vi "stage-field-test.vi"() -> ()   [LabVIEW 2014]
uses:
  stage-controller-globals.vi
panel:
  in  "Z max":dbl=200.0
  out "Current Z (um)":ext
  in  "Current Z 2":ext(slide) scale=-1.0..1.0 scale format="%_3f"
  in  "Field Size":enum16{"0", "1", "4", "9", "16"}(ring)=enum."16"
  in  "Field Number":u32(slide)=6 min=1 max=16 step=1 scale=1.0..16.0
  in  "Stop":bool
  in  "Reset":bool
  out "Current (X,Y)":cluster{ext[], ext[]}[](graph)=[{[100.0], [100.0]}, {[100.0, 150.0], [50.0, 50.0]}, {[100.0, 150.0], [100.0, 100.0]}]
  out "At limit 2":bool
  out "At limit":bool
  out "Current X":dbl=100.0 format="%#_13g"
  out "Current Y":dbl=100.0 format="%#_13g"
  in  "x,y step (um)":ext=10.0 format="%_5g"
  in  "x-":bool=TRUE
  in  "x+":bool=TRUE
  in  "y-":bool=TRUE
  in  "y+":bool=TRUE
  in  "Y max":dbl=200.0
  in  "X max":dbl=200.0
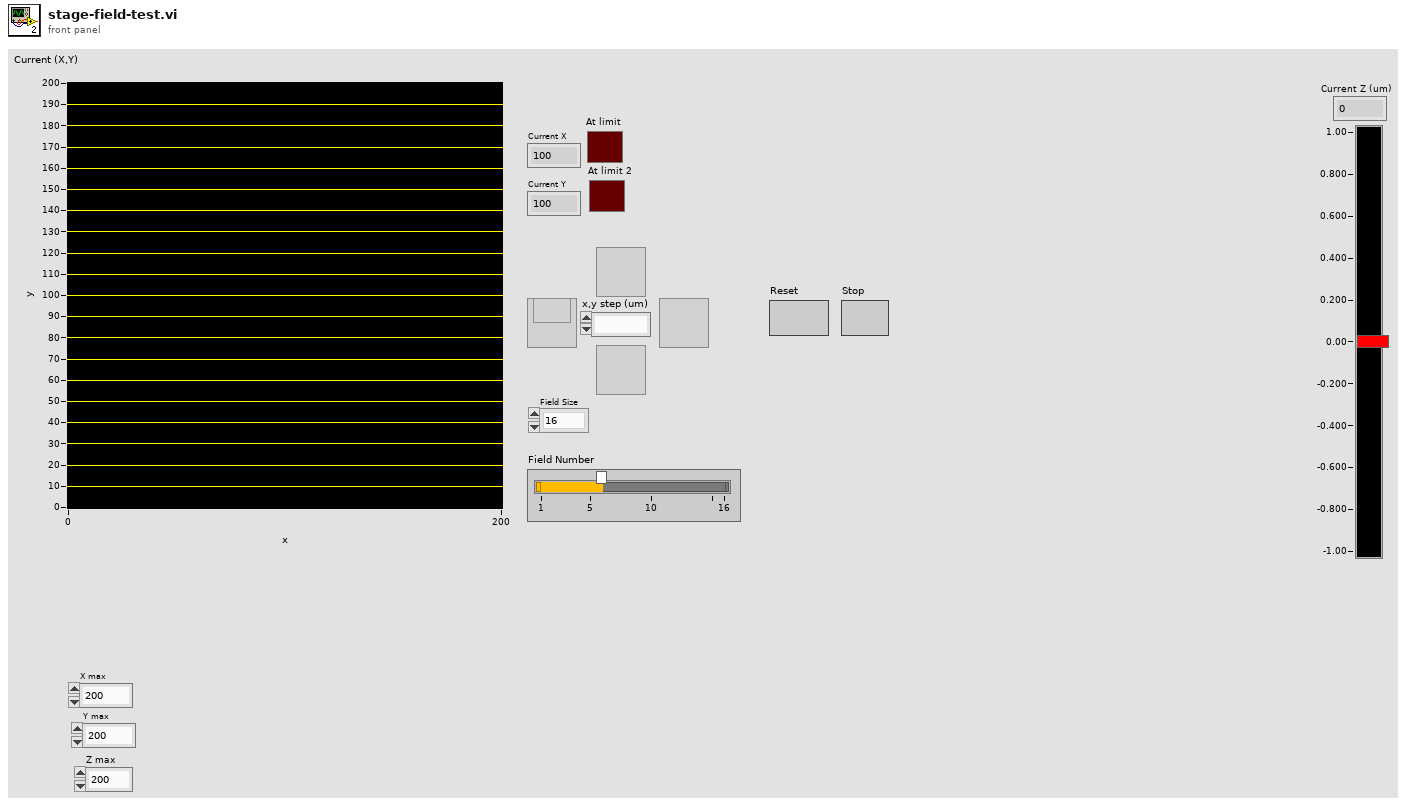
[diagram p1: front panel]
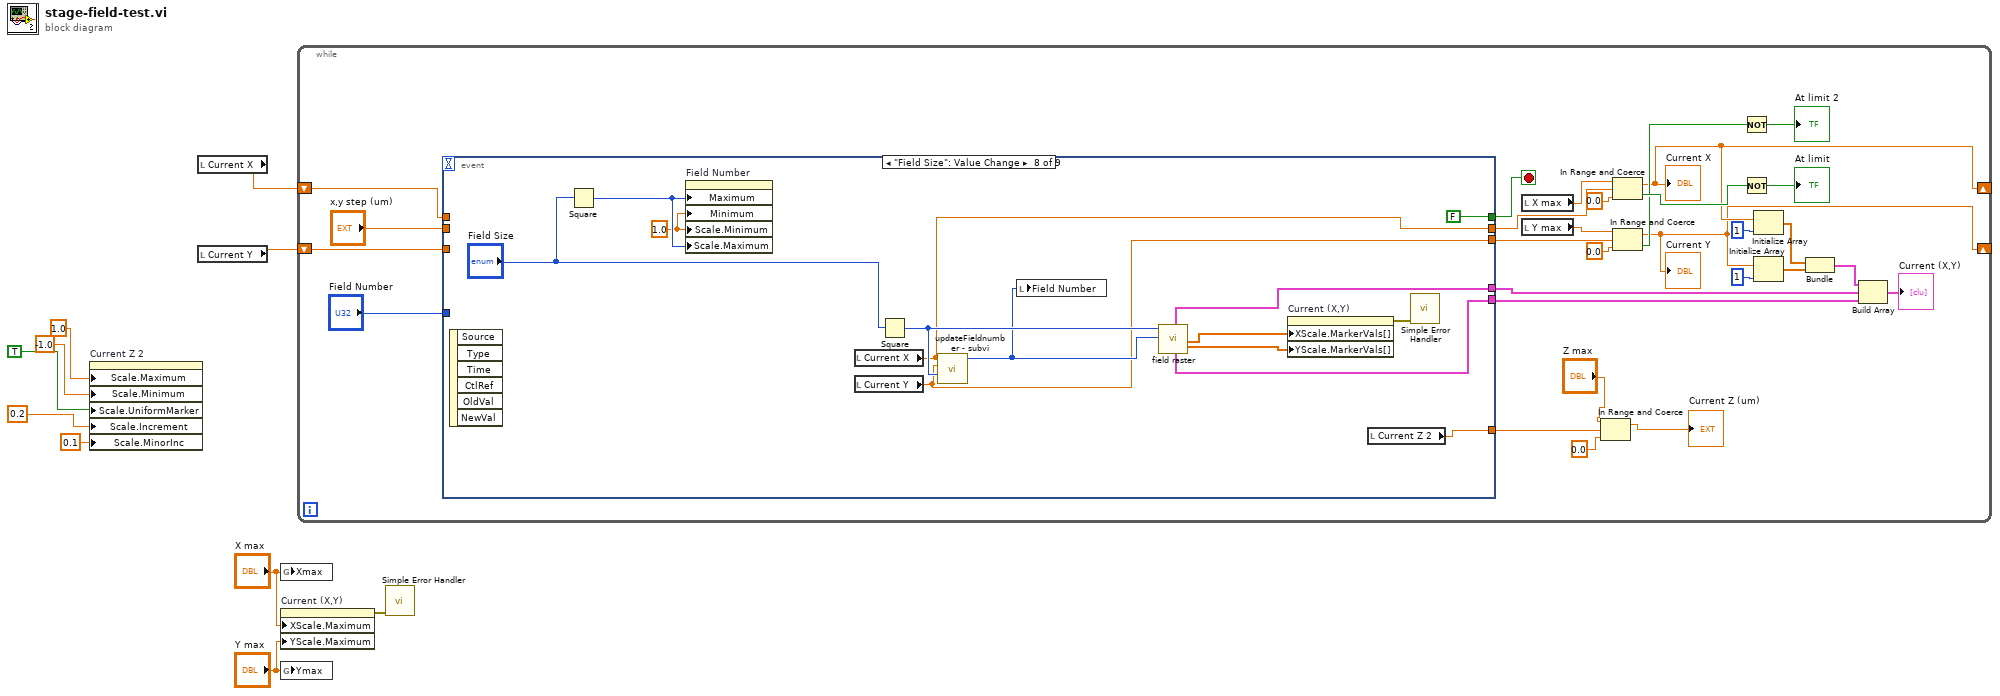
[diagram p0: block diagram]
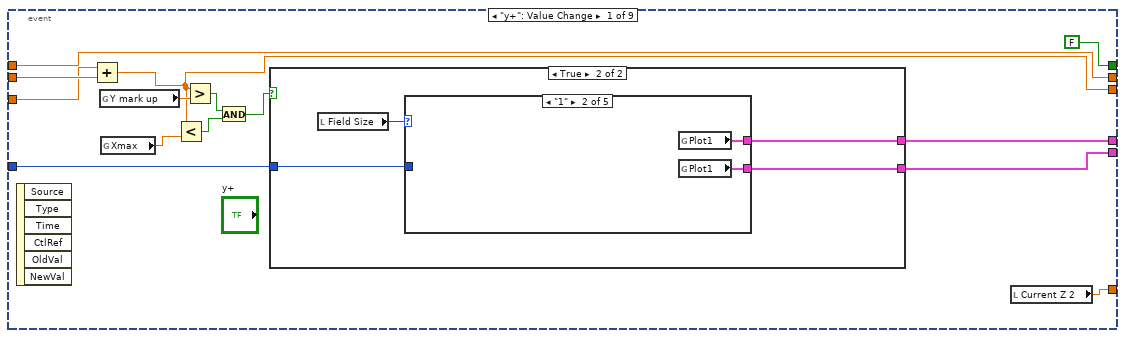
[diagram p2: hidden frame]
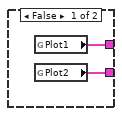
[diagram p3: hidden frame]
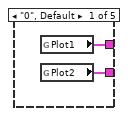
[diagram p4: hidden frame]
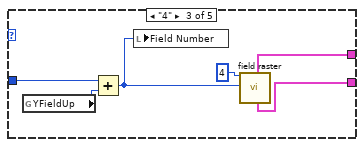
[diagram p5: hidden frame]
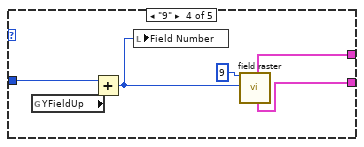
[diagram p6: hidden frame]
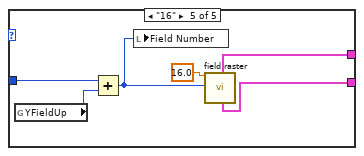
[diagram p7: hidden frame]
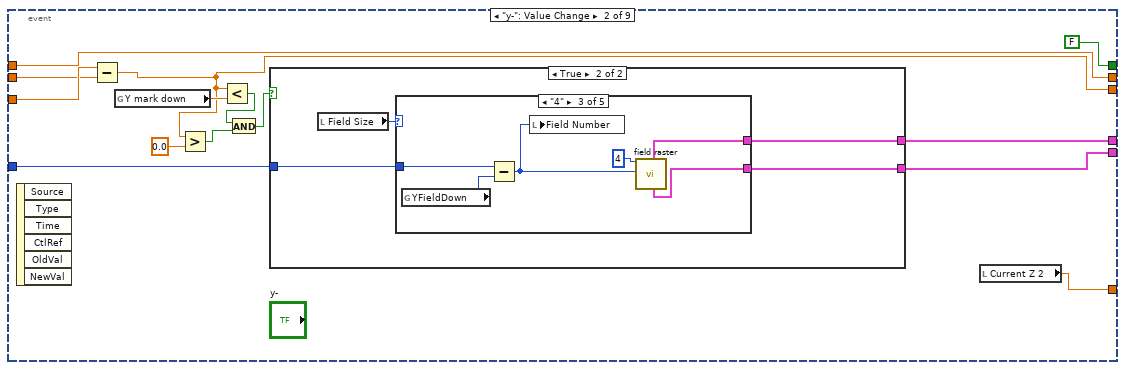
[diagram p8: hidden frame]
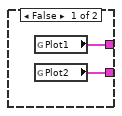
[diagram p9: hidden frame]
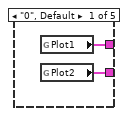
[diagram p10: hidden frame]
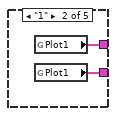
[diagram p11: hidden frame]
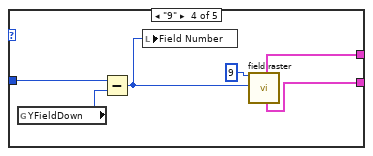
[diagram p12: hidden frame]
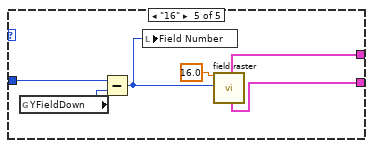
[diagram p13: hidden frame]
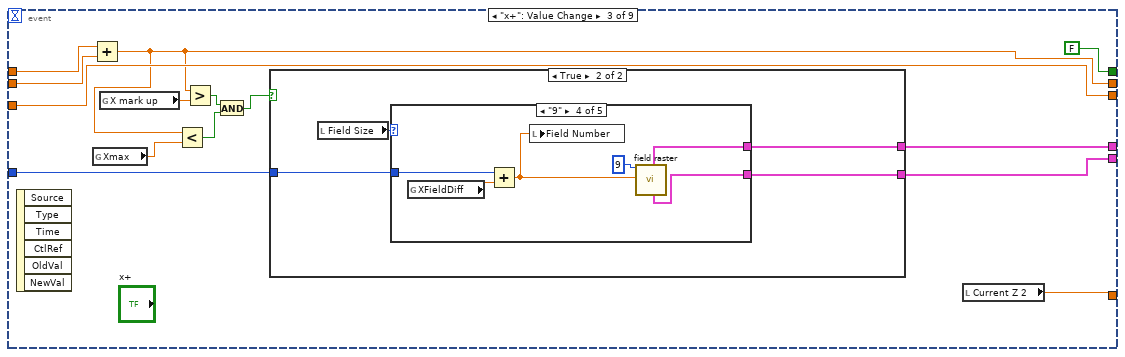
[diagram p14: hidden frame]
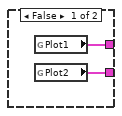
[diagram p15: hidden frame]
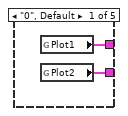
[diagram p16: hidden frame]
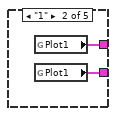
[diagram p17: hidden frame]
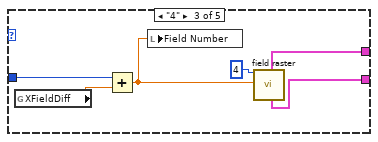
[diagram p18: hidden frame]
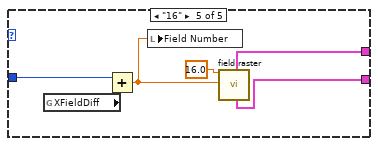
[diagram p19: hidden frame]
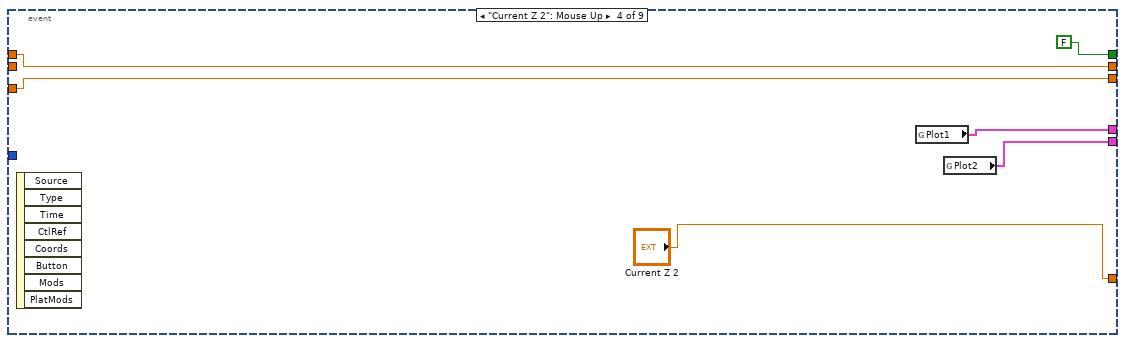
[diagram p20: hidden frame]
diagram:
  n1 = property on="Current Z 2" class="Slide (strict)"("Scale.Maximum"=1.0 ("Scale.Range:Maximum"), "Scale.Minimum"=-1.0 ("Scale.Range:Minimum"), "Scale.UniformMarker"=TRUE, "Scale.Increment"=0.2 ("Scale.Range:Increment"), "Scale.MinorInc"=0.1 ("Scale.Range:Minor Increment")) -> ()  [unwired: 2 in, 2 out]
  n2 = local read "Current X"() -> (w6:dbl)
  n3 = local read "Current Y"() -> (w7:dbl)
  n4 = global write "stage-controller-globals.vi" "Xmax"("X max") -> ()
  n5 = property on="Current (X,Y)" class="XYGraph (strict)"("XScale.Maximum"="X max", "YScale.Maximum"="Y max") -> (error out=w10:errorcluster)  [unwired: 2 in, 1 out]
  n6 = global write "stage-controller-globals.vi" "Ymax"("Y max") -> ()
  n7 = while {
    shift-right: [w27] -> _
    shift-left: w6 -> [w39]
    shift-right: [w26] -> _
    shift-left: w7 -> [w38]
    stop <- w32 stop-if-true
    n8 = event shown="[7] \"Field Size\": Value Change" {
      selector: _ -> [_ _ _ _ _ _ _ _ _]
      dyn-events: _ -> [_ _ _ _ _ _ _ _ _]
      timeout: _ -> [_ _ _ _ _ _ _ _ _]
      tunnel: w39 -> [w43 w84 w137 w170 w185 w218 _ _ _]
      tunnel: w38 -> [w52 w95 w135 w171 w183 w217 _ _ _]
      tunnel: "x,y step (um)" -> [w53 w94 w136 _ w184 _ _ _ _]
      tunnel: [w41 w83 w135 w171 w183 w217 w222 w256 w273] -> w12
      tunnel: [w43 w84 w126 w170 w174 w218 w221 w257 w274] -> w11
      tunnel: [FALSE FALSE FALSE FALSE FALSE "Stop" FALSE FALSE FALSE] -> w32
      tunnel: "Field Number" -> [w49 w90 w131 _ w181 _ _ _ _]
      tunnel: [w48 w91 w132 w167 w178 w216 w224 w265 w271] -> w19
      tunnel: [w47 w92 w133 w168 w179 w215 w223 w264 w272] -> w18
      tunnel: [w40 w82 w124 "Current Z 2" w172 w214 w220 w261 w270] -> w14
      event "y+": Value Change {
        n9 = event-data() -> ()  [unwired: 1 in, 6 out]
        n10 = Add(x=w52, y=w53) -> (x+y=w41:ext)
        n11 = global read "stage-controller-globals.vi" "Y mark up"() -> (w50:dbl)
        n12 = global read "stage-controller-globals.vi" "Xmax"() -> (w42:dbl)
        n13 = Less?(x=w41, y=w42) -> (x < y?=w44:bool)
        n14 = Greater?(x=w41, y=w50) -> (0:w45:bool)
        n15 = And(x=w45, y=w44) -> (x .and. y?=w46:bool)
        n16 = case shown="True" w46 {
          tunnel: w49 -> [_ w58]
          tunnel: [w55 w57] -> w48
          tunnel: [w54 w56] -> w47
          frame False {
            n17 = global read "stage-controller-globals.vi" "Plot1"() -> (w55:cluster{dbl[], dbl[]})
            n18 = global read "stage-controller-globals.vi" "Plot2"() -> (w54:cluster{dbl[], dbl[]})
          }
          frame True {
            n19 = local read "Field Size"() -> (w59:enum16{"0", "1", "4", "9", "16"})
            n20 = case shown="\"1\"" w59 {
              tunnel: w58 -> [_ _ w69 w73 w79]
              tunnel: [w61 w63 w68 w75 w81] -> w57
              tunnel: [w60 w62 w67 w74 w80] -> w56
              frame "0", Default {
                n21 = global read "stage-controller-globals.vi" "Plot1"() -> (w61:cluster{dbl[], dbl[]})
                n22 = global read "stage-controller-globals.vi" "Plot2"() -> (w60:cluster{dbl[], dbl[]})
              }
              frame "1" {
                n23 = global read "stage-controller-globals.vi" "Plot1"() -> (w63:cluster{dbl[], dbl[]})
                n24 = global read "stage-controller-globals.vi" "Plot1"() -> (w62:cluster{dbl[], dbl[]})
              }
              frame "4" {
                n25 = global read "stage-controller-globals.vi" "YFieldUp"() -> (w64:u32)
                n26 = Add(x=w69, y=w64) -> (x+y=w65:u32)
                n27 = local write "Field Number"(w65) -> ()
                n28 = call "field raster.vi"("field size"=4, "field number"=w65) -> ("Plot1"=w68:cluster{dbl[], dbl[]}, "Plot2"=w67:cluster{dbl[], dbl[]})  [unwired: 12 in, 4 out]
              }
              frame "9" {
                n29 = global read "stage-controller-globals.vi" "YFieldUp"() -> (w70:u32)
                n30 = Add(x=w73, y=w70) -> (x+y=w71:u32)
                n31 = local write "Field Number"(w71) -> ()
                n32 = call "field raster.vi"("field size"=9, "field number"=w71) -> ("Plot1"=w75:cluster{dbl[], dbl[]}, "Plot2"=w74:cluster{dbl[], dbl[]})  [unwired: 12 in, 4 out]
              }
              frame "16" {
                n33 = global read "stage-controller-globals.vi" "YFieldUp"() -> (w76:u32)
                n34 = Add(x=w79, y=w76) -> (x+y=w77:u32)
                n35 = local write "Field Number"(w77) -> ()
                n36 = call "field raster.vi"("field size"=16.0, "field number"=w77) -> ("Plot1"=w81:cluster{dbl[], dbl[]}, "Plot2"=w80:cluster{dbl[], dbl[]})  [unwired: 12 in, 4 out]
              }
            }
          }
        }
        n37 = local read "Current Z 2"() -> (w40:ext)
      }
      event "y-": Value Change {
        n38 = event-data() -> ()  [unwired: 1 in, 6 out]
        n39 = Subtract(x=w95, y=w94) -> (x-y=w83:ext)
        n40 = global read "stage-controller-globals.vi" "Y mark down"() -> (w89:dbl)
        n41 = Greater?(x=w83, y=0.0) -> (0:w86:bool)
        n42 = Less?(x=w83, y=w89) -> (x < y?=w87:bool)
        n43 = And(x=w87, y=w86) -> (x .and. y?=w88:bool)
        n44 = case shown="True" w88 {
          tunnel: w90 -> [_ w101]
          tunnel: [w97 w100] -> w91
          tunnel: [w96 w99] -> w92
          frame False {
            n45 = global read "stage-controller-globals.vi" "Plot1"() -> (w97:cluster{dbl[], dbl[]})
            n46 = global read "stage-controller-globals.vi" "Plot2"() -> (w96:cluster{dbl[], dbl[]})
          }
          frame True {
            n47 = local read "Field Size"() -> (w98:enum16{"0", "1", "4", "9", "16"})
            n48 = case shown="\"4\"" w98 {
              tunnel: w101 -> [_ _ w111 w115 w121]
              tunnel: [w103 w105 w110 w117 w123] -> w100
              tunnel: [w102 w104 w109 w116 w122] -> w99
              frame "0", Default {
                n49 = global read "stage-controller-globals.vi" "Plot1"() -> (w103:cluster{dbl[], dbl[]})
                n50 = global read "stage-controller-globals.vi" "Plot2"() -> (w102:cluster{dbl[], dbl[]})
              }
              frame "1" {
                n51 = global read "stage-controller-globals.vi" "Plot1"() -> (w105:cluster{dbl[], dbl[]})
                n52 = global read "stage-controller-globals.vi" "Plot1"() -> (w104:cluster{dbl[], dbl[]})
              }
              frame "4" {
                n53 = global read "stage-controller-globals.vi" "YFieldDown"() -> (w106:u32)
                n54 = Subtract(x=w111, y=w106) -> (x-y=w107:u32)
                n55 = local write "Field Number"(w107) -> ()
                n56 = call "field raster.vi"("field size"=4, "field number"=w107) -> ("Plot1"=w110:cluster{dbl[], dbl[]}, "Plot2"=w109:cluster{dbl[], dbl[]})  [unwired: 12 in, 4 out]
              }
              frame "9" {
                n57 = global read "stage-controller-globals.vi" "YFieldDown"() -> (w112:u32)
                n58 = Subtract(x=w115, y=w112) -> (x-y=w113:u32)
                n59 = local write "Field Number"(w113) -> ()
                n60 = call "field raster.vi"("field size"=9, "field number"=w113) -> ("Plot1"=w117:cluster{dbl[], dbl[]}, "Plot2"=w116:cluster{dbl[], dbl[]})  [unwired: 12 in, 4 out]
              }
              frame "16" {
                n61 = global read "stage-controller-globals.vi" "YFieldDown"() -> (w118:u32)
                n62 = Subtract(x=w121, y=w118) -> (x-y=w119:u32)
                n63 = local write "Field Number"(w119) -> ()
                n64 = call "field raster.vi"("field size"=16.0, "field number"=w119) -> ("Plot1"=w123:cluster{dbl[], dbl[]}, "Plot2"=w122:cluster{dbl[], dbl[]})  [unwired: 12 in, 4 out]
              }
            }
          }
        }
        n65 = local read "Current Z 2"() -> (w82:ext)
      }
      event "x+": Value Change {
        n66 = event-data() -> ()  [unwired: 1 in, 6 out]
        n67 = Add(x=w137, y=w136) -> (x+y=w126:ext)
        n68 = global read "stage-controller-globals.vi" "Xmax"() -> (w125:dbl)
        n69 = global read "stage-controller-globals.vi" "X mark up"() -> (w130:dbl)
        n70 = Less?(x=w126, y=w125) -> (x < y?=w127:bool)
        n71 = Greater?(x=w126, y=w130) -> (0:w129:bool)
        n72 = And(x=w129, y=w127) -> (x .and. y?=w128:bool)
        n73 = case shown="True" w128 {
          tunnel: w131 -> [_ w143]
          tunnel: [w139 w142] -> w132
          tunnel: [w138 w141] -> w133
          frame False {
            n74 = global read "stage-controller-globals.vi" "Plot1"() -> (w139:cluster{dbl[], dbl[]})
            n75 = global read "stage-controller-globals.vi" "Plot2"() -> (w138:cluster{dbl[], dbl[]})
          }
          frame True {
            n76 = local read "Field Size"() -> (w140:enum16{"0", "1", "4", "9", "16"})
            n77 = case shown="\"9\"" w140 {
              tunnel: w143 -> [_ _ w153 w157 w163]
              tunnel: [w145 w147 w152 w159 w165] -> w142
              tunnel: [w144 w146 w151 w158 w164] -> w141
              frame "0", Default {
                n78 = global read "stage-controller-globals.vi" "Plot1"() -> (w145:cluster{dbl[], dbl[]})
                n79 = global read "stage-controller-globals.vi" "Plot2"() -> (w144:cluster{dbl[], dbl[]})
              }
              frame "1" {
                n80 = global read "stage-controller-globals.vi" "Plot1"() -> (w147:cluster{dbl[], dbl[]})
                n81 = global read "stage-controller-globals.vi" "Plot1"() -> (w146:cluster{dbl[], dbl[]})
              }
              frame "4" {
                n82 = global read "stage-controller-globals.vi" "XFieldDiff"() -> (w148:dbl)
                n83 = Add(x=w153, y=w148) -> (x+y=w149:dbl)
                n84 = local write "Field Number"(w149) -> ()
                n85 = call "field raster.vi"("field size"=4, "field number"=w149) -> ("Plot1"=w152:cluster{dbl[], dbl[]}, "Plot2"=w151:cluster{dbl[], dbl[]})  [unwired: 12 in, 4 out]
              }
              frame "9" {
                n86 = global read "stage-controller-globals.vi" "XFieldDiff"() -> (w154:dbl)
                n87 = Add(x=w157, y=w154) -> (x+y=w155:dbl)
                n88 = local write "Field Number"(w155) -> ()
                n89 = call "field raster.vi"("field size"=9, "field number"=w155) -> ("Plot1"=w159:cluster{dbl[], dbl[]}, "Plot2"=w158:cluster{dbl[], dbl[]})  [unwired: 12 in, 4 out]
              }
              frame "16" {
                n90 = global read "stage-controller-globals.vi" "XFieldDiff"() -> (w160:dbl)
                n91 = Add(x=w163, y=w160) -> (x+y=w161:dbl)
                n92 = local write "Field Number"(w161) -> ()
                n93 = call "field raster.vi"("field size"=16.0, "field number"=w161) -> ("Plot1"=w165:cluster{dbl[], dbl[]}, "Plot2"=w164:cluster{dbl[], dbl[]})  [unwired: 12 in, 4 out]
              }
            }
          }
        }
        n94 = local read "Current Z 2"() -> (w124:ext)
      }
      event "Current Z 2": Mouse Up {
        n95 = event-data() -> ()  [unwired: 1 in, 8 out]
        n96 = global read "stage-controller-globals.vi" "Plot1"() -> (w167:cluster{dbl[], dbl[]})
        n97 = global read "stage-controller-globals.vi" "Plot2"() -> (w168:cluster{dbl[], dbl[]})
      }
      event "x-": Value Change {
        n98 = event-data() -> ()  [unwired: 1 in, 6 out]
        n99 = Subtract(x=w185, y=w184) -> (x-y=w174:ext)
        n100 = global read "stage-controller-globals.vi" "X mark down"() -> (w180:dbl)
        n101 = Greater?(x=w174, y=ext 0.0) -> (0:w175:bool)
        n102 = Less?(x=w174, y=w180) -> (x < y?=w177:bool)
        n103 = And(x=w177, y=w175) -> (x .and. y?=w176:bool)
        n104 = case shown="True" w176 {
          tunnel: w181 -> [_ w191]
          tunnel: [w187 w190] -> w178
          tunnel: [w186 w189] -> w179
          frame False {
            n105 = global read "stage-controller-globals.vi" "Plot1"() -> (w187:cluster{dbl[], dbl[]})
            n106 = global read "stage-controller-globals.vi" "Plot2"() -> (w186:cluster{dbl[], dbl[]})
          }
          frame True {
            n107 = local read "Field Size"() -> (w188:enum16{"0", "1", "4", "9", "16"})
            n108 = case shown="\"4\"" w188 {
              tunnel: w191 -> [_ _ w201 w205 w211]
              tunnel: [w193 w195 w200 w207 w213] -> w190
              tunnel: [w192 w194 w199 w206 w212] -> w189
              frame "0", Default {
                n109 = global read "stage-controller-globals.vi" "Plot1"() -> (w193:cluster{dbl[], dbl[]})
                n110 = global read "stage-controller-globals.vi" "Plot2"() -> (w192:cluster{dbl[], dbl[]})
              }
              frame "1" {
                n111 = global read "stage-controller-globals.vi" "Plot1"() -> (w195:cluster{dbl[], dbl[]})
                n112 = global read "stage-controller-globals.vi" "Plot1"() -> (w194:cluster{dbl[], dbl[]})
              }
              frame "4" {
                n113 = global read "stage-controller-globals.vi" "XFieldDiff"() -> (w196:dbl)
                n114 = Subtract(x=w201, y=w196) -> (x-y=w197:dbl)
                n115 = local write "Field Number"(w197) -> ()
                n116 = call "field raster.vi"("field size"=4, "field number"=w197) -> ("Plot1"=w200:cluster{dbl[], dbl[]}, "Plot2"=w199:cluster{dbl[], dbl[]})  [unwired: 12 in, 4 out]
              }
              frame "9" {
                n117 = global read "stage-controller-globals.vi" "XFieldDiff"() -> (w202:dbl)
                n118 = Subtract(x=w205, y=w202) -> (x-y=w203:dbl)
                n119 = local write "Field Number"(w203) -> ()
                n120 = call "field raster.vi"("field size"=9, "field number"=w203) -> ("Plot1"=w207:cluster{dbl[], dbl[]}, "Plot2"=w206:cluster{dbl[], dbl[]})  [unwired: 12 in, 4 out]
              }
              frame "16" {
                n121 = global read "stage-controller-globals.vi" "XFieldDiff"() -> (w208:dbl)
                n122 = Subtract(x=w211, y=w208) -> (x-y=w209:dbl)
                n123 = local write "Field Number"(w209) -> ()
                n124 = call "field raster.vi"("field size"=16.0, "field number"=w209) -> ("Plot1"=w213:cluster{dbl[], dbl[]}, "Plot2"=w212:cluster{dbl[], dbl[]})  [unwired: 12 in, 4 out]
              }
            }
          }
        }
        n125 = local read "Current Z 2"() -> (w172:ext)
      }
      event "Stop": Value Change {
        n126 = event-data() -> ()  [unwired: 1 in, 6 out]
        n127 = local read "Current Z 2"() -> (w214:ext)
        n128 = global read "stage-controller-globals.vi" "Plot1"() -> (w216:cluster{dbl[], dbl[]})
        n129 = global read "stage-controller-globals.vi" "Plot2"() -> (w215:cluster{dbl[], dbl[]})
      }
      event "Reset": Value Change {
        n130 = event-data() -> ()  [unwired: 1 in, 6 out]
        n131 = local read "Field Size"() -> (w225:enum16{"0", "1", "4", "9", "16"})
        n132 = case shown="\"16\"" w225 {
          selector: w225 -> [_ w233 _ _ _]
          tunnel: [w228 w235 _ w244 w250] -> w224
          tunnel: [w229 w234 _ w243 w249] -> w223
          tunnel: [w227 w231 w240 w242 w253] -> w222
          tunnel: [w227 w230 w239 w241 w252] -> w221
          frame "0", Default {
            w227 = 0.0
            n133 = global read "stage-controller-globals.vi" "Plot1"() -> (w228:cluster{dbl[], dbl[]})
            n134 = global read "stage-controller-globals.vi" "Plot2"() -> (w229:cluster{dbl[], dbl[]})
          }
          frame "1" {
            n135 = call "field raster.vi"("field size"=w233, "field number"=1) -> ("Plot1"=w235:cluster{dbl[], dbl[]}, "Plot2"=w234:cluster{dbl[], dbl[]}, "current Y"=w230:dbl, "current X"=w231:dbl)  [unwired: 12 in, 2 out]
          }
          frame "4" {
            w238 = 2
            n136 = global read "stage-controller-globals.vi" "Xmax"() -> (w237:dbl)
            n137 = global read "stage-controller-globals.vi" "Ymax"() -> (w236:dbl)
            n138 = Divide(x=w237, y=w238) -> (x/y=w239:dbl)
            n139 = Divide(x=w236, y=w238) -> (x/y=w240:dbl)
          }
          frame "9" {
            w245 = 5
            n140 = local write "Field Number"(w245) -> ()
            n141 = call "field raster.vi"("field size"=9, "field number"=w245) -> ("Plot1"=w244:cluster{dbl[], dbl[]}, "Plot2"=w243:cluster{dbl[], dbl[]}, "current Y"=w241:dbl, "current X"=w242:dbl)  [unwired: 12 in, 2 out]
          }
          frame "16" {
            w248 = 2
            w247 = 6
            n142 = local write "Field Number"(w247) -> ()
            n143 = global read "stage-controller-globals.vi" "Xmax"() -> (w254:dbl)
            n144 = global read "stage-controller-globals.vi" "Ymax"() -> (w255:dbl)
            n145 = call "field raster.vi"("field size"=16, "field number"=w247) -> ("Plot1"=w250:cluster{dbl[], dbl[]}, "Plot2"=w249:cluster{dbl[], dbl[]})  [unwired: 12 in, 4 out]
            n146 = Divide(x=w254, y=w248) -> (x/y=w252:dbl)
            n147 = Divide(x=w255, y=w248) -> (x/y=w253:dbl)
          }
        }
        n148 = local read "Current Z 2"() -> (w220:ext)
      }
      event "Field Size": Value Change {
        w259 = 1.0
        n149 = event-data() -> ()  [unwired: 1 in, 6 out]
        n150 = Square(x="Field Size") -> (x^2=w260:u16)
        n151 = property on="Field Number" class="Slide (strict)"("Maximum"=w260, "Minimum"=w259, "Scale.Minimum"=w259, "Scale.Maximum"=w260) -> ()  [unwired: 2 in, 2 out]
        n152 = local read "Current X"() -> (w257:dbl)
        n153 = local read "Current Y"() -> (w256:dbl)
        n154 = Square(x="Field Size") -> (x^2=w263:u16)
        n155 = call "updateFieldnumber - subvi.vi"("Field Size"=w263, "CurY"=w256, "CurX"=w257) -> ("Field Number"=w262:u32)  [unwired: 8 in]
        n156 = local write "Field Number"(w262) -> ()
        n157 = call "field raster.vi"("field size"=w263, "field number"=w262) -> ("Plot1"=w265:cluster{dbl[], dbl[]}, "Plot2"=w264:cluster{dbl[], dbl[]}, "x mark"=w267:dbl[], "y mark"=w269:dbl[])  [unwired: 12 in, 2 out]
        n158 = property on="Current (X,Y)" class="XYGraph (strict)"("XScale.MarkerVals[]"=w267, "YScale.MarkerVals[]"=w269) -> (error out=w268:errorcluster)  [unwired: 2 in, 1 out]
        n159 = local read "Current Z 2"() -> (w261:ext)
        n160 = call <vilib>:"Simple Error Handler.vi"("error in (no error)"=w268) -> ()  [unwired: 4 in, 5 out]
      }
      event "Field Number": Value Change {
        n161 = event-data() -> ()  [unwired: 1 in, 6 out]
        n162 = local read "Field Size"() -> (w275:enum16{"0", "1", "4", "9", "16"})
        n163 = local read "Field Number"() -> (w278:u32)
        n164 = Square(x=w275) -> (x^2=w276:u16)
        n165 = local read "Current Z 2"() -> (w270:ext)
        n166 = call "field raster.vi"("field size"=w276, "field number"=w278) -> ("Plot1"=w271:cluster{dbl[], dbl[]}, "Plot2"=w272:cluster{dbl[], dbl[]}, "current Y"=w274:dbl, "current X"=w273:dbl)  [unwired: 12 in, 2 out]
      }
    }
    n167 = local read "X max"() -> (w35:dbl)
    n168 = local read "Y max"() -> (w33:dbl)
    n169 = In Range and Coerce(upper limit="Z max", x=w14, lower limit=0.0) -> (coerced(x)=→"Current Z (um)":ext)  [unwired: 1 out]
    n170 = In Range and Coerce(upper limit=w35, x=w11, lower limit=0.0) -> (coerced(x)=w27:ext, In Range?=w31:bool)
    "Current X" <- w27
    n171 = In Range and Coerce(upper limit=w33, x=w12, lower limit=0.0) -> (coerced(x)=w26:ext, In Range?=w30:bool)
    "Current Y" <- w26
    n172 = Not(x=w30) -> (.not. x?=→"At limit 2":bool)
    n173 = Not(x=w31) -> (.not. x?=→"At limit":bool)
    n174 = Initialize Array(w27, 1) -> (w22:ext[])
    n175 = Initialize Array(w26, 1) -> (w23:ext[])
    n176 = Bundle(w22, w23) -> (w20:cluster{ext[], ext[]})  [unwired: 1 out]
    n177 = Build Array(w20, w19, w18) -> (→"Current (X,Y)":cluster{ext[], ext[]}[])
  }
  n178 = call <vilib>:"Simple Error Handler.vi"("error in (no error)"=w10) -> ()  [unwired: 4 in, 5 out]
